vi "Match Meta.vi"(8 "error in (no error)":errorcluster, 9 "Value (Any)":string=".", 10 "Name":string, 11 "Config Lookup (New)":refnum<class "Config Lookup.lvclass">) -> (0 "error out":errorcluster, 3 "Config Lookup out":refnum<class "Config Lookup.lvclass">)   [LabVIEW 2020, in "CDM-Config.lvlib" / "Config Lookup.lvclass"]
doc: "Adds a Meta field that must be matched when performing lookups within the config. If <b>Value</b> is unspecified then the element just needs to have a meta field that matches the specified name otherwise it must also match the value.\n\nValue is matched using the <b>Match Pattern</b> node which also provides basic regular expression matching."
uses:
  Config Filter/Config Lookup.lvclass
  Meta Data.ctl
  Config Filter/Config Lookup.lvclass/Config Lookup.ctl
  CDM-Config.lvlib
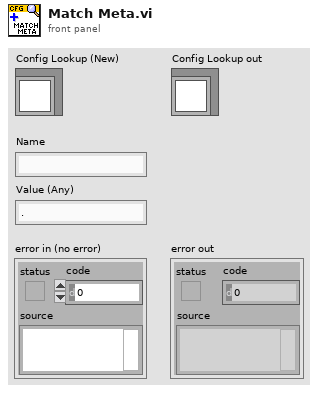
[diagram p1: front panel]
types:
  T1 = typedef "CDM-Config.lvlib/Meta Data.ctl" = cluster{"Name":string, "Value":string}
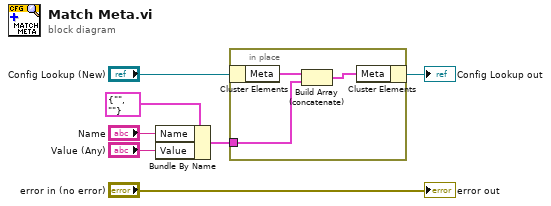
[diagram p0: block diagram]
diagram:
  n1 = Bundle By Name(cluster=T1 {"Name"="", "Value"=""} ("Meta Data"), "Name"="Name", "Value"="Value (Any)") -> (w2:T1)
  n2 = in-place {
    in-place-border: w2 -> [w9]
    n3 = in-place-cluster #1("Config Lookup (New)") -> ("Meta"=w10:T1[])
    n4 = Build Array (concatenate)(w10, w9) -> (w8:T1[])
    n5 = in-place-cluster #1("Meta"=w8) -> (→"Config Lookup out":refnum<class "Config Lookup.lvclass">)
  }
  "error out" <- "error in (no error)"
